vi "Index of Call.vi"(6 "Comparator":refnum<class "Comparator.lvclass">, 8 "error in (no error)":errorcluster, 10 "VI Call":refnum<class "VI Call.lvclass">, 11 "Unique Calls":refnum<class "VI Call.lvclass">[](array[class])) -> (0 "error out":errorcluster, 3 "f":i32)   [LabVIEW 2020, in "Never.lvlib" / "Never.lvclass"]
uses:
  Never.lvclass
  Core/VI Call/VI Call.lvclass
  Core/Comparator/Comparator.lvclass
  Never.lvclass/Never.ctl
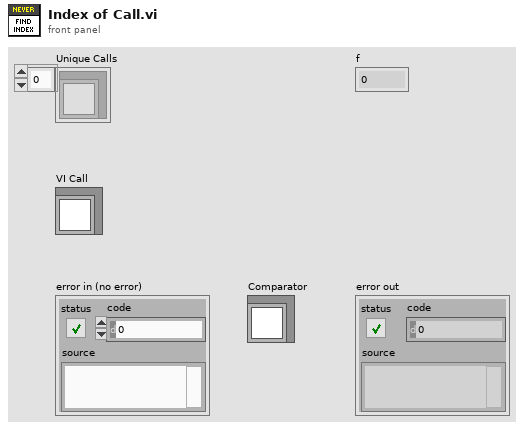
[diagram p1: front panel]
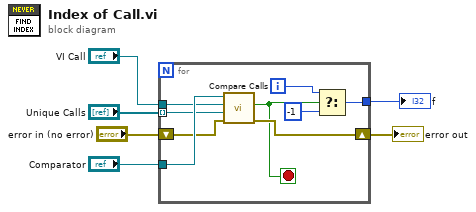
[diagram p0: block diagram]
diagram:
  n1 = for {
    tunnel: "Comparator" -> [w15]
    tunnel: "VI Call" -> [w14]
    tunnel: "Unique Calls" -> [w13] mode=indexing
    shift-right: [w11] -> w5
    shift-left: "error in (no error)" -> [w12]
    tunnel: [w7] -> w6
    i -> [w9]
    stop <- w10 stop-if-true
    n2 = call-dynamic "Compare Calls.vi"("error in (no error)"=w12, "VI Call 2"=w13, "VI Call 1"=w14, "Comparator in"=w15) -> ("error out"=w11:errorcluster, "Equal?"=w10:bool)  [unwired: 5 in, 1 out]
    n3 = Select(t=w9, s=w10, f=-1) -> (s? t:f=w7:i32)
  }
  "f" <- w6
  "error out" <- w5
